vi "Matrix_read_target.vi"() -> ()   [LabVIEW 2013]
uses:
  <vilib>/Platform/TimedLoop/XDataNode/timing_clust.ctl
  <vilib>/Platform/TimedLoop/XDataNode/nitl_modes.ctl
  <vilib>/Platform/TimedLoop/XDataNode/wakeup.ctl
  <vilib>/rvi/Emulation/niFpgaSctlEmulationGetInTimedLoop.vi
  <vilib>/rvi/Emulation/niFpgaEmulationReportErrorSimple.vi
  <vilib>/rvi/Emulation/niFpgaGetClockAttributes.vi
  <vilib>/rvi/Emulation/niFpgaCriticalErrorInLSC.vi
  <vilib>/rvi/eio/common/nirviEmuTemplateMethod_errors.vi
  <vilib>/Platform/TimedLoop/XDataNode/XDataNode.xnode
  <vilib>/eio/EIONode/EIONode.xnode
  <vilib>/Platform/TimedLoop/XDataNode/XDNodeRunTimeDep.lvlib
panel:
  in  "1_EXTCLK_divider":i16=1
  in  "Write2":bool=TRUE
  in  "Write1":bool=TRUE
  in  "WE1":bool=TRUE
  in  "WE2":bool=TRUE
  in  "89":i16=89
  in  "72":i16=72
  in  "71":i16=71
  in  "53":i16=53
  in  "100_Sclk_divider":i32=100
  in  "0_WE_counter":i32
  in  "50_Fall/Rise_counter":i32=50
  in  "Read2":u8 format="%x"
  in  "Read1":u8 format="%x"
  in  "Device_Read":u8=187 format="%x"
  in  "Reg":u8=9 format="%x"
  in  "Device_Write":u8=186 format="%x"
  in  "35":i16=35
  in  "17":i16=17
  in  "36":i16=36
  in  "18":i16=18
  # "!!!11111!!!!"
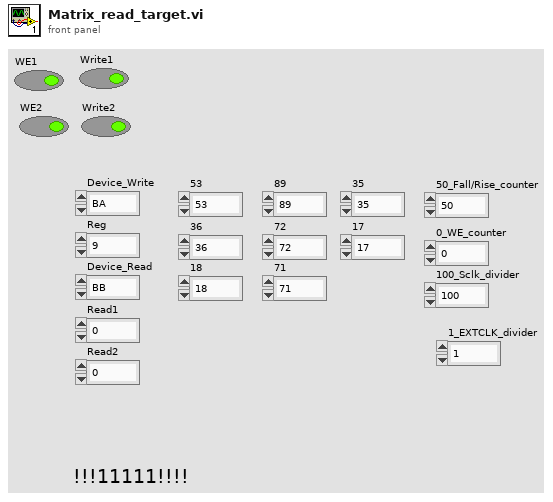
[diagram p1: front panel]
types:
  T1 = typedef "XDNodeRunTimeDep.lvlib/timing_clust.ctl" = cluster{"Expected End [f-1]":u64, "Actual End [f-1]":u64, "Finished Late? [f-1]":bool, "Expected End [i-1]":u64, "Actual End [i-1]":u64, "Finished Late? [i-1]":bool, "Expected Start [i]":u64, "Actual Start [i]":u64, "Expected Start [f]":u64, "Actual Start [f]":u64, "Source Name":string, "Structure Name":string, "Period":i64, "Deadline":i64, "Offset":i64, "Start":i64, "Priority":i32, "Timeout":i32, "Mode":T2, "Wakeup Reason":T3, "Error":errorcluster, "Source Type":string, "Secondary Source Type":string, "Global End Time":u64, "Global Start Time":u64, "Frame Duration":u64, "Iteration Duration":u64, "Assigned CPU":i32, "I/O Scan Engine Mode":u32}
  T2 = typedef "XDNodeRunTimeDep.lvlib/nitl_modes.ctl" = enum32{"No Change", "Process missed periods, maintain original phase", "Discard missed periods, maintain original phase", "Process missed periods, ignore original phase", "Discard missed periods, ignore original phase"}
  T3 = typedef "XDNodeRunTimeDep.lvlib/wakeup.ctl" = enum32{"Normal", "Aborted", "Asynchronous wakeup", "Timing source error", "Timed loop error", "Timeout"}
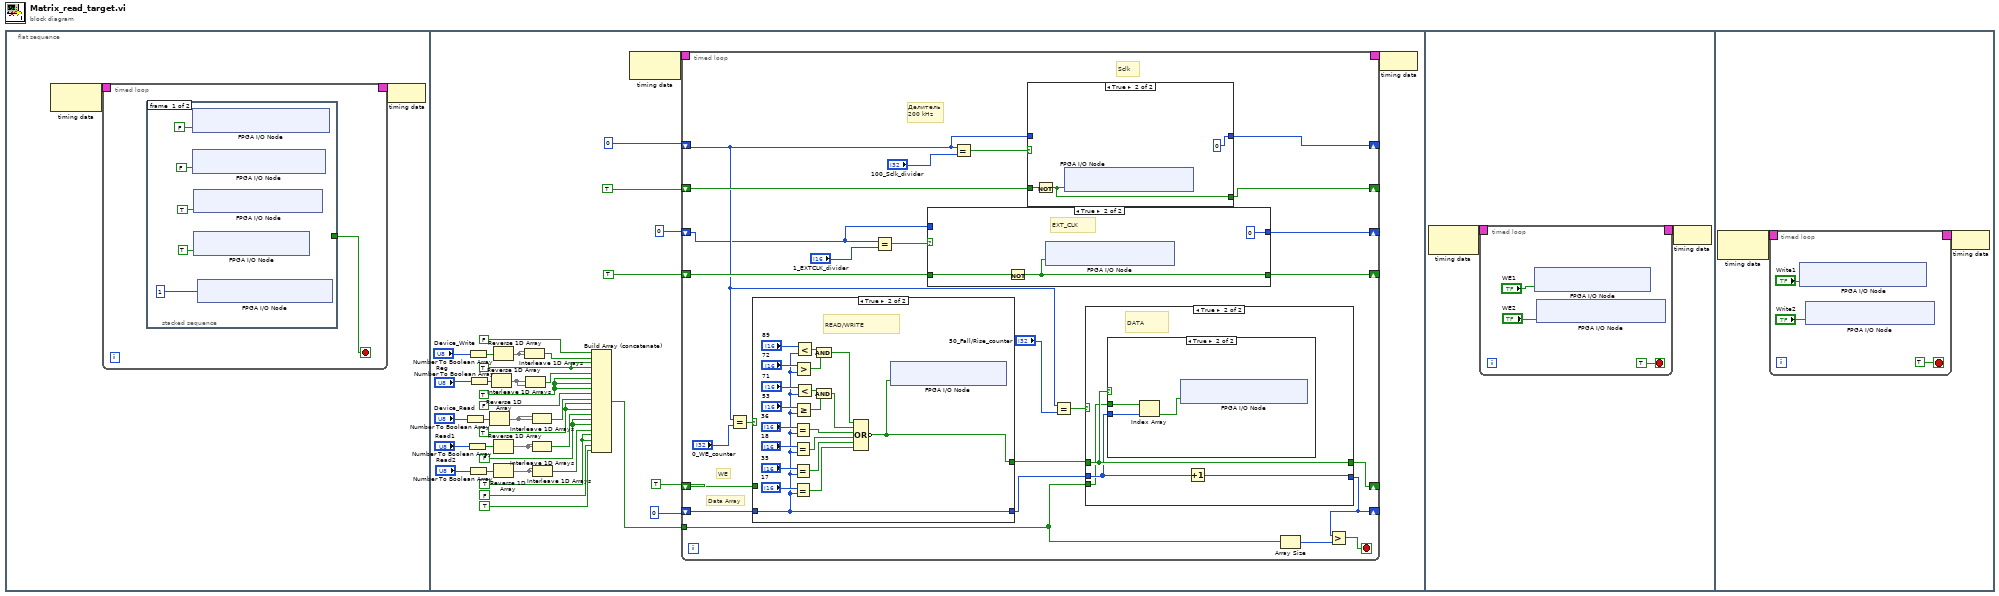
[diagram p0: block diagram]
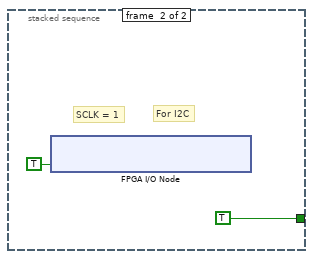
[diagram p2: hidden frame]
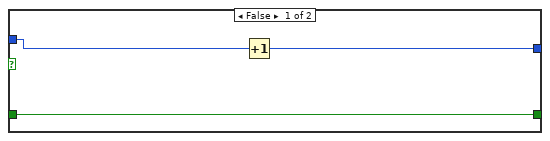
[diagram p3: hidden frame]
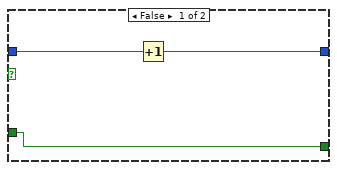
[diagram p7: hidden frame]
diagram:
  n1 = flat-sequence {
    frame #0 {
      n2 = node-c288() -> (w2:T1)  [unwired: 1 in]
      n3 = timed-loop {
        timing: w2 -> [_]
        timing-out: [_] -> w1
        stop <- w3 stop-if-true
        n4 = stacked-sequence {
          tunnel: [_ TRUE] -> w3
          frame #0 {
            n5 = xnode "FPGA I/O Node"("IO Module\\DDCA_DIO16-23_WE"=FALSE ("IO Module\\DDCA_DIO16-23_WE")) -> ()  [unwired: 1 in, 1 out]
            n6 = xnode "FPGA I/O Node"("IO Module\\DDCA_DIO8-15_WE"=FALSE ("IO Module\\DDCA_DIO8-15_WE")) -> ()  [unwired: 1 in, 1 out]
            n7 = xnode "FPGA I/O Node"("IO Module\\DDCA_DIO0-7_WE"=TRUE ("IO Module\\DDCA_DIO0-7_WE")) -> ()  [unwired: 1 in, 1 out]
            n8 = xnode "FPGA I/O Node"("IO Module\\DDCA_PFI_WE"=TRUE ("IO Module\\DDCA_DIO0-7_WE")) -> ()  [unwired: 1 in, 1 out]
            n9 = xnode "FPGA I/O Node"("IO Module\\Local_Supply_Select"=u8 1 ("IO Module\\Local_Supply_Select")) -> ()  [unwired: 1 in, 1 out]
          }
          frame #1 {
            # "For I2C"
            # "SCLK = 1"
            n10 = xnode "FPGA I/O Node"("IO Module\\DDCA_DIO6_Write"=TRUE ("IO Module\\DDCA_DIO6_Write")) -> ()  [unwired: 1 in, 1 out]
          }
        }
      }
      n11 = node-c288(w1) -> ()
    }
    frame #1 {
      w25 = TRUE
      w27 = FALSE
      w31 = TRUE
      w34 = TRUE
      w37 = TRUE
      n12 = Number To Boolean Array(number="Device_Read") -> (Boolean array=w42:bool[])
      n13 = Number To Boolean Array(number="Read1") -> (Boolean array=w22:bool[])
      n14 = Number To Boolean Array(number="Device_Write") -> (Boolean array=w40:bool[])
      n15 = Number To Boolean Array(number="Read2") -> (Boolean array=w21:bool[])
      n16 = Number To Boolean Array(number="Reg") -> (Boolean array=w41:bool[])
      n17 = Reverse 1D Array(array=w42) -> (reversed array=w18:bool[])
      n18 = Reverse 1D Array(array=w41) -> (reversed array=w19:bool[])
      n19 = Reverse 1D Array(array=w40) -> (reversed array=w20:bool[])
      n20 = Reverse 1D Array(array=w22) -> (reversed array=w17:bool[])
      n21 = Reverse 1D Array(array=w21) -> (reversed array=w16:bool[])
      n22 = Interleave 1D Arrays(w20, w20) -> (w38:bool[])
      n23 = Interleave 1D Arrays(w19, w19) -> (w36:bool[])
      n24 = Interleave 1D Arrays(w18, w18) -> (w32:bool[])
      n25 = Interleave 1D Arrays(w17, w17) -> (w28:bool[])
      n26 = Interleave 1D Arrays(w16, w16) -> (w26:bool[])
      n27 = Build Array (concatenate)(FALSE, w38, w37, w37, w36, w34, w34, w34, FALSE, w32, w31, w31, w28, w27, w27, w26, w25, w25, FALSE, TRUE) -> (w35:bool[])
      n28 = node-c288() -> (w52:T1)  [unwired: 1 in]
      n29 = timed-loop {
        timing: w52 -> [_]
        timing-out: [_] -> w51
        shift-right: [w73] -> _
        shift-left: i16 0 -> [w63]
        shift-right: [w74] -> _
        shift-left: TRUE -> [w75]
        shift-right: [w71] -> _
        shift-left: TRUE -> [w72]
        shift-right: [w68] -> _
        shift-left: TRUE -> [w70]
        shift-right: [w58] -> _
        shift-left: i16 0 -> [w62]
        tunnel: w35 -> [w60]
        shift-right: [w53] -> _
        shift-left: i16 0 -> [w54]
        stop <- w59 stop-if-true
        # "Data Array"
        # "WE"
        # "Sclk"
        # "Делитель\n200 kHz"
        n30 = Equal?(x=w63, y="0_WE_counter") -> (x = y?=w67:bool)
        n31 = case shown="True" w67 {
          tunnel: [w85 w101] -> w69
          tunnel: w70 -> [w85 _]
          tunnel: w62 -> [w84 w87]
          tunnel: [w84 w87] -> w61
          frame False {
          }
          frame True {
            # "READ/WRITE"
            n32 = Equal?(x="36", y=w87) -> (x = y?=w97:bool)
            n33 = Equal?(x="18", y=w87) -> (x = y?=w98:bool)
            n34 = Equal?(x="35", y=w87) -> (x = y?=w103:bool)
            n35 = Equal?(x="17", y=w87) -> (x = y?=w105:bool)
            n36 = Greater?(x="72", y=w87) -> (0:w91:bool)
            n37 = Greater Or Equal?(x="53", y=w87) -> (x >= y?=w93:bool)
            n38 = Less?(x="89", y=w87) -> (x < y?=w90:bool)
            n39 = Less?(x="71", y=w87) -> (x < y?=w94:bool)
            n40 = And(x=w90, y=w91) -> (x .and. y?=w86:bool)
            n41 = And(x=w94, y=w93) -> (x .and. y?=w92:bool)
            n42 = Compound Arithmetic op=OR(w86, w92, w97, w98, w103, w105) -> (invert w101:bool)
            n43 = xnode "FPGA I/O Node"("IO Module\\DDCA_PFI_WE"=w101) -> ()  [unwired: 1 in, 1 out]
          }
        }
        n44 = Equal?(x=w54, y="1_EXTCLK_divider") -> (x = y?=w56:bool)
        n45 = case shown="True" w56 {
          tunnel: w72 -> [w79 w83]
          tunnel: [w79 w82] -> w71
          tunnel: w54 -> [w80 _]
          tunnel: [w78 i16 0] -> w53
          frame False {
            n46 = Increment(x=w80) -> (x+1=w78:i16)
          }
          frame True {
            # "EXT_CLK"
            n47 = Not(x=w83) -> (.not. x?=w82:bool)
            n48 = xnode "FPGA I/O Node"("IO Module\\DDCA_DIO7_Write"=w82) -> ()  [unwired: 1 in, 1 out]
          }
        }
        n49 = Equal?(x=w63, y="100_Sclk_divider") -> (x = y?=w77:bool)
        n50 = case shown="True" w77 {
          tunnel: [w117 0] -> w73
          tunnel: w75 -> [w116 w119]
          tunnel: [w116 w118] -> w74
          tunnel: w63 -> [w115 _]
          frame False {
            n51 = Increment(x=w115) -> (x+1=w117:i32)
          }
          frame True {
            n52 = Not(x=w119) -> (.not. x?=w118:bool)
            n53 = xnode "FPGA I/O Node"("IO Module\\DDCA_DIO6_Write"=w118) -> ()  [unwired: 1 in, 1 out]
          }
        }
        n54 = Equal?(x=w63, y="50_Fall/Rise_counter") -> (x = y?=w64:bool)
        n55 = case shown="True" w64 {
          tunnel: w69 -> [w107 w111]
          tunnel: [w107 w111] -> w68
          tunnel: w61 -> [w106 w110]
          tunnel: [w106 w109] -> w58
          tunnel: w60 -> [_ w108]
          frame False {
          }
          frame True {
            # "DATA"
            n56 = case shown="True" w111 {
              tunnel: w110 -> [_ w114]
              tunnel: w108 -> [_ w113]
              frame False {
              }
              frame True {
                n57 = Index Array(array=w113, index=w114) -> (element=w112:bool)
                n58 = xnode "FPGA I/O Node"("IO Module\\DDCA_PFI1_Write"=w112) -> ()  [unwired: 1 in, 1 out]
              }
            }
            n59 = Increment(x=w110) -> (x+1=w109:i16)
          }
        }
        n60 = Array Size(array=w60) -> (size(s)=w57:i32)
        n61 = Greater?(x=w58, y=w57) -> (0:w59:bool)
      }
      n62 = node-c288(w51) -> ()
    }
    frame #2 {
      n63 = node-c288() -> (w126:T1)  [unwired: 1 in]
      n64 = timed-loop {
        timing: w126 -> [_]
        timing-out: [_] -> w125
        stop <- TRUE stop-if-true
        n65 = xnode "FPGA I/O Node"("IO Module\\DDCA_PFI_WE"="WE1") -> ()  [unwired: 1 in, 1 out]
        n66 = xnode "FPGA I/O Node"("IO Module\\DDCA_DIO0-7_WE"="WE2") -> ()  [unwired: 1 in, 1 out]
      }
      n67 = node-c288(w125) -> ()
    }
    frame #3 {
      n68 = node-c288() -> (w135:T1)  [unwired: 1 in]
      n69 = timed-loop {
        timing: w135 -> [_]
        timing-out: [_] -> w134
        stop <- TRUE stop-if-true
        n70 = xnode "FPGA I/O Node"("IO Module\\DDCA_PFI1_Write"="Write1") -> ()  [unwired: 1 in, 1 out]
        n71 = xnode "FPGA I/O Node"("IO Module\\DDCA_DIO6_Write"="Write2") -> ()  [unwired: 1 in, 1 out]
      }
      n72 = node-c288(w134) -> ()
    }
  }
